vi "Vecto Node.vi"(8 "error in (no error)":errorcluster, 11 "Node in":refnum<class "Node Config.lvclass">) -> (0 "error out":errorcluster, 2 "Vecto Node":refnum<class "Node Config.lvclass">, 3 "Node out":refnum<class "Node Config.lvclass">)   [LabVIEW 2020, in "VolatusConfig.lvlib" / "Node Config.lvclass"]
uses:
  Node Config.lvclass
  Node Config.lvclass/Node Config.ctl
  VolatusConfigElement/VolatusConfigElement.lvclass
  Cluster/Cluster Config.lvclass
  lv-vecto/Vecto/Node Config/Node Config.lvclass
  lv-vecto/Vecto/Node Config/Node Info.ctl
  lv-vecto/VectoConfig/VectoConfig.lvlib
  lv-cdm/CDM-Config/Config Filter/Config Lookup.lvclass
  lv-cdm/CDM-Config/Config Element/Config Element.lvclass
  Meta Name.ctl
  VolatusConfig.lvlib
  C:/dev/lv20CE/relink/lv-volatus/VolatusConfig/VolatusConfigElement/VolatusConfigElement.lvclass
  C:/dev/lv20CE/relink/lv-volatus/VolatusConfig/Node/Node Config.lvclass
  C:/dev/lv20CE/relink/lv-volatus/VolatusConfig/Cluster/Cluster Config.lvclass
  System/System Config.lvclass
  C:/dev/lv20CE/relink/lv-volatus/VolatusConfig/System/System Config.lvclass
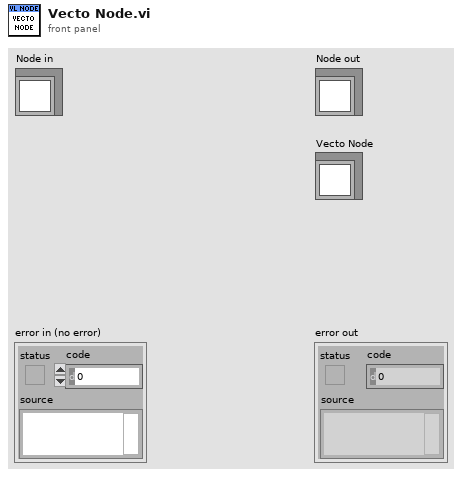
[diagram p1: front panel]
types:
  T1 = typedef "VolatusConfig.lvlib/Meta Name.ctl" = enum16{"VL_Type", "VL_Node_IP", "VL_Node_Type", "VL_Task_Type", "VL_Group_Type", "VL_Channel_Type", "VL_Channel_DataType", "VL_Config_Version", "VL_Overlay_Type", "VL_Config_Hash"}
  T2 = typedef "VectoConfig.lvlib/Node Info.ctl" = cluster{"System":string, "Cluster":string, "Name":string, "ID":u32, "Capabilities":string[]}
  T3 = typedef "VectoConfig.lvlib/Target Group Info.ctl" = cluster{"Name":string, "ID":u32, "Nodes":T4[]}
  T4 = typedef "VectoConfig.lvlib/Node Name ID.ctl" = cluster{"Name":string, "ID":u32}
  T5 = typedef "VectoConfig.lvlib/Telemetry Config.ctl" = cluster{"Routing":T6, "Endpoint":T7}
  T6 = typedef "VectoConfig.lvlib/Telemetry Routing.ctl" = enum16{"Multicast", "Unicast"}
  T7 = typedef "VectoConfig.lvlib/Endpoint.ctl" = cluster{"Address":string, "Port":u16}
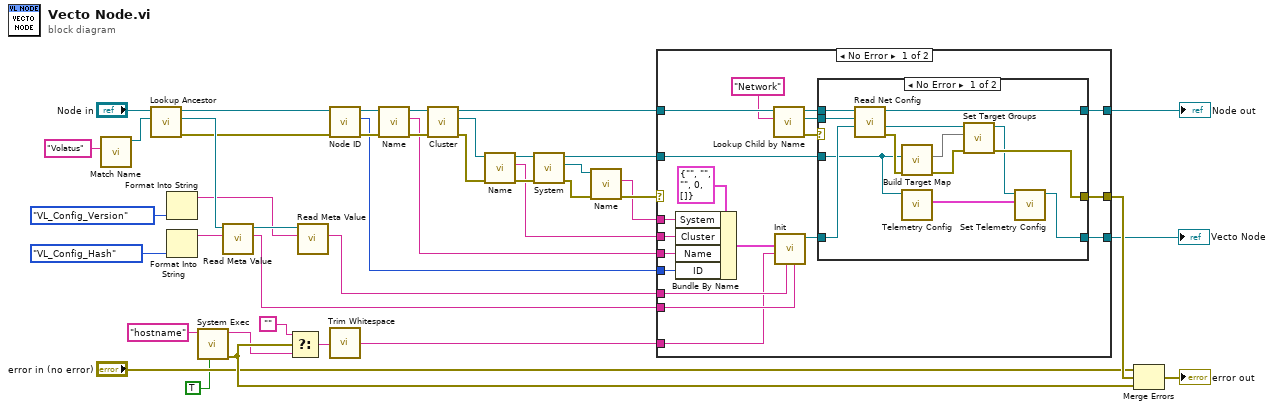
[diagram p0: block diagram]
diagram:
  n1 = call "Match Name.vi"("Name"="Volatus") -> ("Config Lookup out"=w16:refnum<class "Config Lookup.lvclass">)  [unwired: 9 in, 1 out]
  n2 = call "Lookup Ancestor.vi"("Lookup"=w16, "VolatusConfigElement in"="Node in") -> ("error out"=w7:errorcluster, "Ancestor"=w13:refnum<class "Config Element.lvclass">, "VolatusConfigElement out"=w18:refnum<class "Node Config.lvclass">)  [unwired: 7 in]
  n3 = Format Into String(Meta_Name."VL_Config_Version" ("Meta Name")) -> (resulting string=w9:string)  [unwired: 3 in, 1 out]
  n4 = Format Into String(Meta_Name."VL_Config_Hash" ("Meta Name")) -> (resulting string=w15:string)  [unwired: 3 in, 1 out]
  n5 = call <vilib>:"System Exec.vi"("run minimized? (F)"=TRUE, "command line"="hostname") -> ("error out"=w42:errorcluster, "standard output"=w5:string)  [unwired: 6 in, 2 out]
  n6 = call "Read Meta Value.vi"("Meta Name"=w15, "Config Element in"=w13) -> ("Meta Value"=w12:string, "Config Element out"=w10:refnum<class "Config Element.lvclass">)  [unwired: 7 in, 1 out]
  n7 = Select(t="", s=w42, f=w5) -> (s? t:f=w3:string)
  n8 = call "Read Meta Value.vi"("Meta Name"=w9, "Config Element in"=w10) -> ("Meta Value"=w8:string)  [unwired: 7 in, 2 out]
  n9 = call "Node ID.vi"("error in (no error)"=w7, "Node in"=w18) -> ("error out"=w25:errorcluster, "Node ID"=w24:u32, "Node out"=w26:refnum<class "Node Config.lvclass">)  [unwired: 7 in]
  n10 = call <vilib>:"Trim Whitespace.vi"("string"=w3) -> ("trimmed string"=w2:string)  [unwired: 1 in]
  n11 = call "Name.vi"("error in (no error)"=w25, "VolatusConfigElement in"=w26) -> ("error out"=w33:errorcluster, "Name"=w27:string, "VolatusConfigElement out"=w37:refnum<class "Node Config.lvclass">)  [unwired: 7 in]
  n12 = call "Cluster.vi"("error in (no error)"=w33, "Node in"=w37) -> ("error out"=w32:errorcluster, "Cluster"=w36:refnum<class "Cluster Config.lvclass">, "Node out"=w38:refnum<class "Node Config.lvclass">)  [unwired: 7 in]
  n13 = call "Name.vi"("error in (no error)"=w32, "VolatusConfigElement in"=w36) -> ("error out"=w31:errorcluster, "Name"=w28:string, "VolatusConfigElement out"=w35:refnum<class "Cluster Config.lvclass">)  [unwired: 7 in]
  n14 = call "System.vi"("error in (no error)"=w31, "Cluster in"=w35) -> ("error out"=w30:errorcluster, "System"=w34:refnum<class "System Config.lvclass">, "Cluster out"=w23:refnum<class "Cluster Config.lvclass">)  [unwired: 7 in]
  n15 = call "Name.vi"("error in (no error)"=w30, "VolatusConfigElement in"=w34) -> ("error out"=w40:errorcluster, "Name"=w29:string)  [unwired: 7 in, 1 out]
  n16 = case shown="No Error" w40 {
    selector: w40 -> [_ w77]
    tunnel: w38 -> [w61 w78]
    tunnel: w29 -> [w58 _]
    tunnel: w28 -> [w57 _]
    tunnel: w27 -> [w56 _]
    tunnel: w24 -> [w55 _]
    tunnel: w23 -> [w47 _]
    tunnel: [w49 w78] -> w22
    tunnel: [w48 _] -> w21
    tunnel: [w46 w77] -> w41
    tunnel: w12 -> [w45 _]
    tunnel: w8 -> [w44 _]
    tunnel: w2 -> [w43 _]
    frame No Error {
      n17 = Bundle By Name(cluster=T2 {"System"="", "Cluster"="", "Name"="", "ID"=0, "Capabilities"=[]} ("Node Info"), "System"=w58, "Cluster"=w57, "Name"=w56, "ID"=w55) -> (w59:T2)
      n18 = call "Lookup Child by Name.vi"("Child Name"="Network", "VolatusConfigElement in"=w61) -> ("error out"=w51:errorcluster, "Child"=w52:refnum<class "Config Element.lvclass">, "VolatusConfigElement out"=w50:refnum<class "Node Config.lvclass">)  [unwired: 6 in, 1 out]
      n19 = call "Init.vi"("Config Hash"=w45, "Config Version"=w44, "Alias (None)"=w43, "Node Info"=w59) -> ("Node out"=w54:refnum<class "Node Config.lvclass">)  [unwired: 6 in, 1 out]
      n20 = case shown="No Error" w51 {
        tunnel: w54 -> [w71 w75]
        tunnel: w52 -> [w72 _]
        tunnel: w50 -> [w73 w76]
        tunnel: [w66 w76] -> w49
        tunnel: [w63 w75] -> w48
        tunnel: w47 -> [w62 _]
        tunnel: [w67 _] -> w46
        frame No Error {
          n21 = call "Read Net Config.vi"("Node Config in"=w71, "Config Element in"=w72, "Node in"=w73) -> ("error out"=w74:errorcluster, "Node Config out"=w70:refnum<class "Node Config.lvclass">, "Node out"=w66:refnum<class "Node Config.lvclass">)  [unwired: 6 in]
          n22 = call "Build Target Map.vi"("error in (no error)"=w74, "Cluster in"=w62) -> ("error out"=w68:errorcluster, "Target Groups"=w69:map{string, T3})  [unwired: 8 in]
          n23 = call "Telemetry Config.vi"("Cluster Config in"=w62) -> ("Telemetry Config"=w65:T5)  [unwired: 8 in, 2 out]
          n24 = call "Set Target Groups.vi"("error in (no error)"=w68, "Target Groups"=w69, "Node Config in"=w70) -> ("error out"=w67:errorcluster, "Node Config out"=w64:refnum<class "Node Config.lvclass">)  [unwired: 7 in]
          n25 = call "Set Telemetry Config.vi"("Telemtry Config"=w65, "Node Config in"=w64) -> ("Node Config out"=w63:refnum<class "Node Config.lvclass">)  [unwired: 8 in, 1 out]
        }
        frame Error {
          # "Networking is optional"
        }
      }
    }
    frame Error {
    }
  }
  "Node out" <- w22
  "Vecto Node" <- w21
  n26 = Merge Errors("error in (no error)", w41, w42) -> (→"error out":errorcluster)
